vi "Add Heat State FGV.vi"(1 "FGV Function":enum16{"Clear", "Set", "Read"}(ring)) -> (0 "Boolean Indicator":bool)   [LabVIEW 2012]
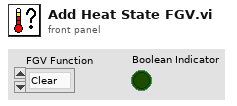
[diagram p1: front panel]
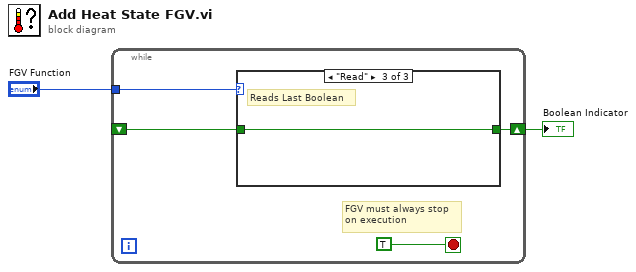
[diagram p0: block diagram]
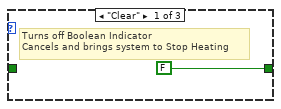
[diagram p2: hidden frame]
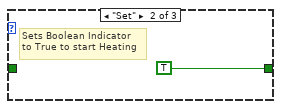
[diagram p3: hidden frame]
diagram:
  n1 = while {
    tunnel: "FGV Function" -> [w6]
    shift-right: [w4] -> w1
    shift-left: _ -> [w3]
    stop <- TRUE stop-if-true
    # "FGV must always stop\non execution"
    n2 = case shown="\"Read\"" w6 {
      tunnel: [FALSE TRUE w9] -> w4
      tunnel: w3 -> [_ _ w9]
      frame "Clear" {
        # "Turns off Boolean Indicator\nCancels and brings system to Stop Heating"
      }
      frame "Set" {
        # "Sets Boolean Indicator \nto True to start Heating"
      }
      frame "Read" {
        # "Reads Last Boolean"
      }
    }
  }
  "Boolean Indicator" <- w1
